vi "Write Vehicle Position.vi"(8 "error in (no error)":errorcluster, 10 "Vehicle Position Simulation":u8(slide) scale=0.0..4.0, 11 "Vehicle Position Simulation Actor in":refnum<class "Vehicle Position Simulation Actor.lvclass">) -> (0 "error out":errorcluster, 3 "Vehicle Position Simulation Actor out":refnum<class "Vehicle Position Simulation Actor.lvclass">)   [LabVIEW 2019, in "Vehicle Position Sinmulation Actor.lvlib" / "Vehicle Position Simulation Actor.lvclass"]
uses:
  Vehicle Position Simulation Actor.lvclass
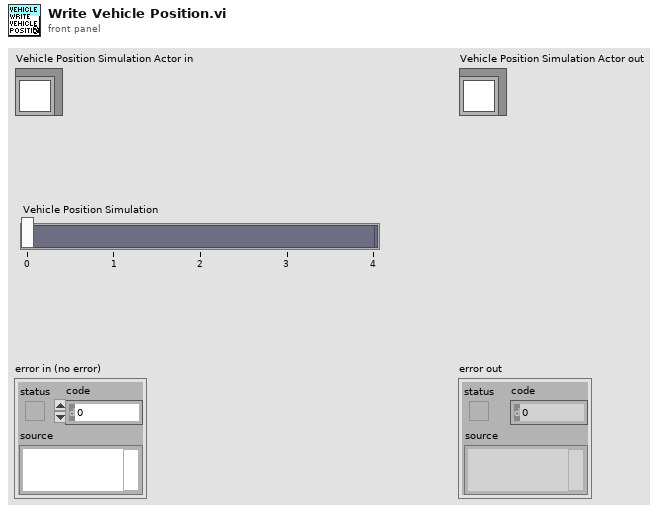
[diagram p1: front panel]
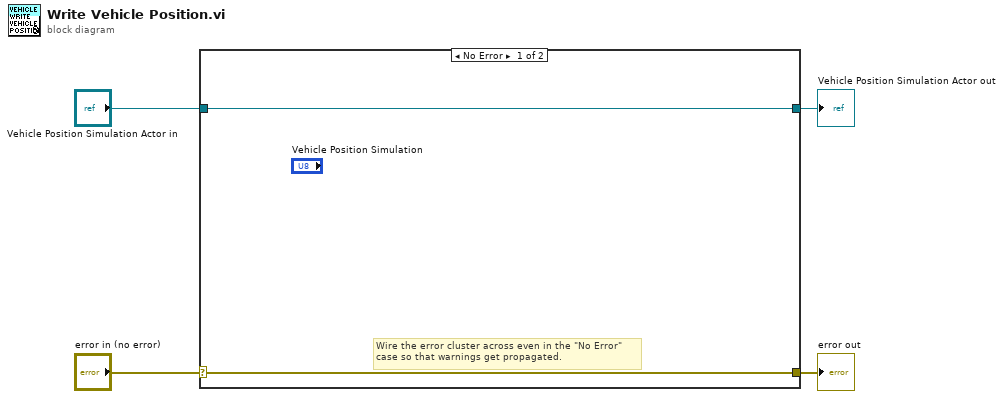
[diagram p0: block diagram]
diagram:
  n1 = case shown="No Error" "error in (no error)" {
    selector: "error in (no error)" -> [w5 w8]
    tunnel: [w5 w8] -> w3
    tunnel: [w6 w7] -> w1
    tunnel: "Vehicle Position Simulation Actor in" -> [w6 w7]
    frame No Error {
      # "Wire the error cluster across even in the \"No Error\"\ncase so that warnings get propagated."
    }
    frame Error {
    }
  }
  "error out" <- w3
  "Vehicle Position Simulation Actor out" <- w1
